vi "Locate P2t.vi"(4 "Template File Path (Locate P2 Hole)":path=path "C:/Users/serce/Desktop/Smart Vision System Testbench/P2/P2 Hole Template.png", 6 "Error In":errorcluster, 9 "Image In":T1) -> (0 "Error Out":errorcluster, 1 "Bounding Box":cluster{"x":sgl, "y":sgl}[](array[cluster]), 3 "Image Out":T1, 5 "Number of Matches (Locate P2 Hole)":i32)   [LabVIEW 2020]
uses:
  <vilib>/vision/Image Controls.llb/IMAQ Image.ctl
  <vilib>/vision/Pattern Matching.llb/IMAQ Curve Parameters.ctl
  <vilib>/vision/Pattern Matching.llb/IMAQ Match Range Setting.ctl
  <vilib>/vision/Pattern Matching.llb/IMAQ Geometric Pattern 2 Advanced Match Options.ctl
  <vilib>/vision/Image Controls.llb/Vision Info Type2.ctl
  <vilib>/vision/NI_Vision_Development_Module.lvlib
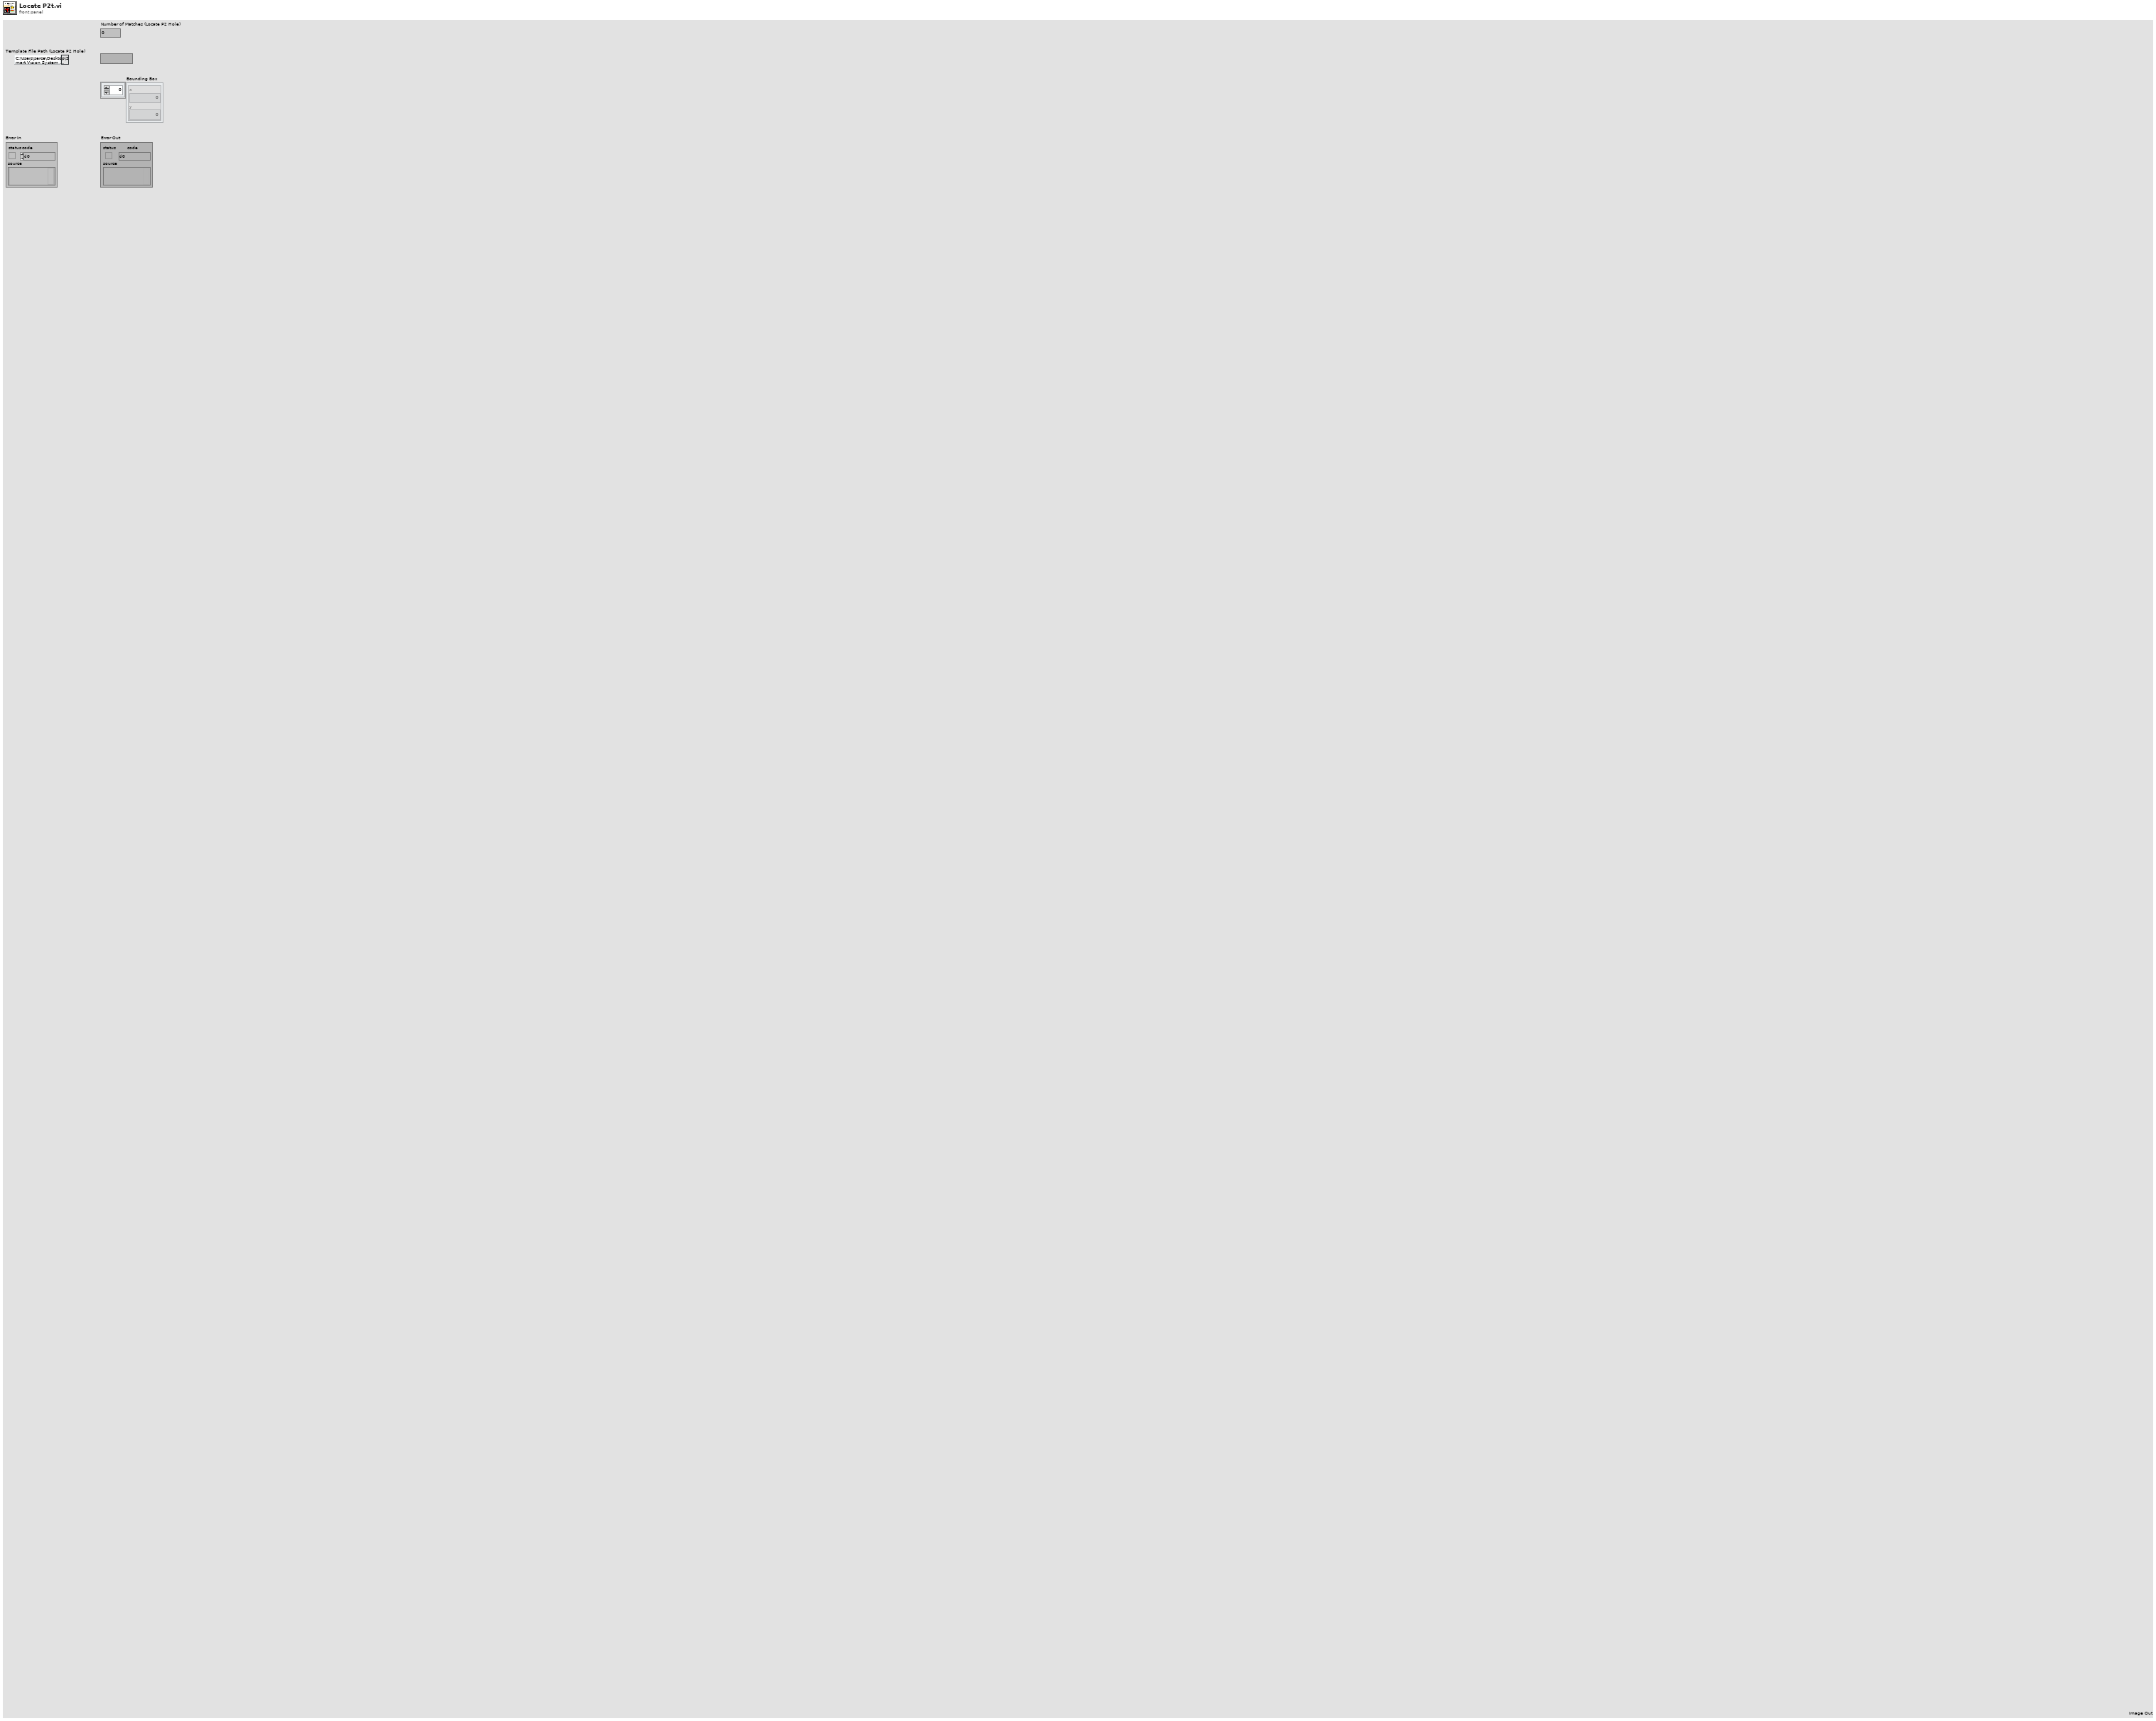
[diagram p1: front panel]
types:
  T1 = typedef "IMAQ Image.ctl" = refnum<image>
  T2 = cluster{"Origin Pixel":cluster{"X":sgl, "Y":sgl}, "X Axis Pixel":cluster{"X":sgl, "Y":sgl}, "Axis Reference":u32}
  T3 = typedef "Vision Info Type2.ctl" = u32
  T4 = typedef "Simple Grid Descriptor" = cluster{"X Step":sgl, "Y Step":sgl, "Unit":T5}
  T5 = typedef "Image Unit" = enum32{"Undefined", "Angström", "Micrometer", "Millimeter", "Centimeter", "Meter", "Kilometer", "Microinch", "Inch", "Feet", "Nautical miles", "Standard miles", "Steps"}
  T6 = enum16{"Reset", "Update Coordinate System", "Get Coordinate System"}
  T7 = enum16{"Horizontal Motion", "Vertical Motion", "Horizontal and Vertical Motion", "Horizontal, Vertical and Angular Motion"}
  T8 = cluster{"Origin":cluster{"X":sgl, "Y":sgl}, "Angle (deg)":sgl, "Axis Reference":u32}
  T9 = typedef "IMAQ Curve Parameters.ctl" = cluster{"Extraction Mode":u32, "Edge Threshold":i32, "Edge Filter Size":u32, "Min Length":i32, "Row Search Step Size":i32, "Col Search Step Size":i32, "Max Endpoint Gap":i32, "Closed":bool, "Subpixel":bool}
  T10 = typedef "IMAQ Match Range Setting.ctl" = cluster{"Match Constraints":u32, "Min":dbl, "Max":dbl}
  T11 = typedef "IMAQ Geometric Pattern 2 Advanced Match Options.ctl" = u16
  T12 = cluster{"Curve Parameters":T9, "Match Mode":cluster{"Rotation":bool, "Scale":bool, "Occlusion":bool, "Reserved 1":bool, "Reserved 2":bool, "Reserved 3":bool}, "Range Settings":T10[], "Number of Matches":i32, "Minimum Match Score":sgl, "SubPixel Accuracy":bool, "Adv. Geometric Match Options 2":cluster{"Setup Data Item":T11, "Item Value":dbl}[]}
  T13 = cluster{"Global Rectangle":i32[], "Contours":cluster{"ID":enum32{"External", "Internal"}, "Type":u32, "Coordinates":i32[]}[]}
  T14 = cluster{"Brightness":sgl, "Contrast":sgl, "Gamma":sgl}
  T15 = typedef "IMAQ GM Match Report.ctl" = cluster{"Position":cluster{"x":sgl, "y":sgl}, "Angle":sgl, "Scale":sgl, "Score":sgl, "Bounding Box":cluster{"x":sgl, "y":sgl}[], "Contrast Reversed":bool, "Occlusion %":sgl, "Template Target Curve Score":sgl, "Target Template Curve Score":sgl, "Correlation Score":sgl}
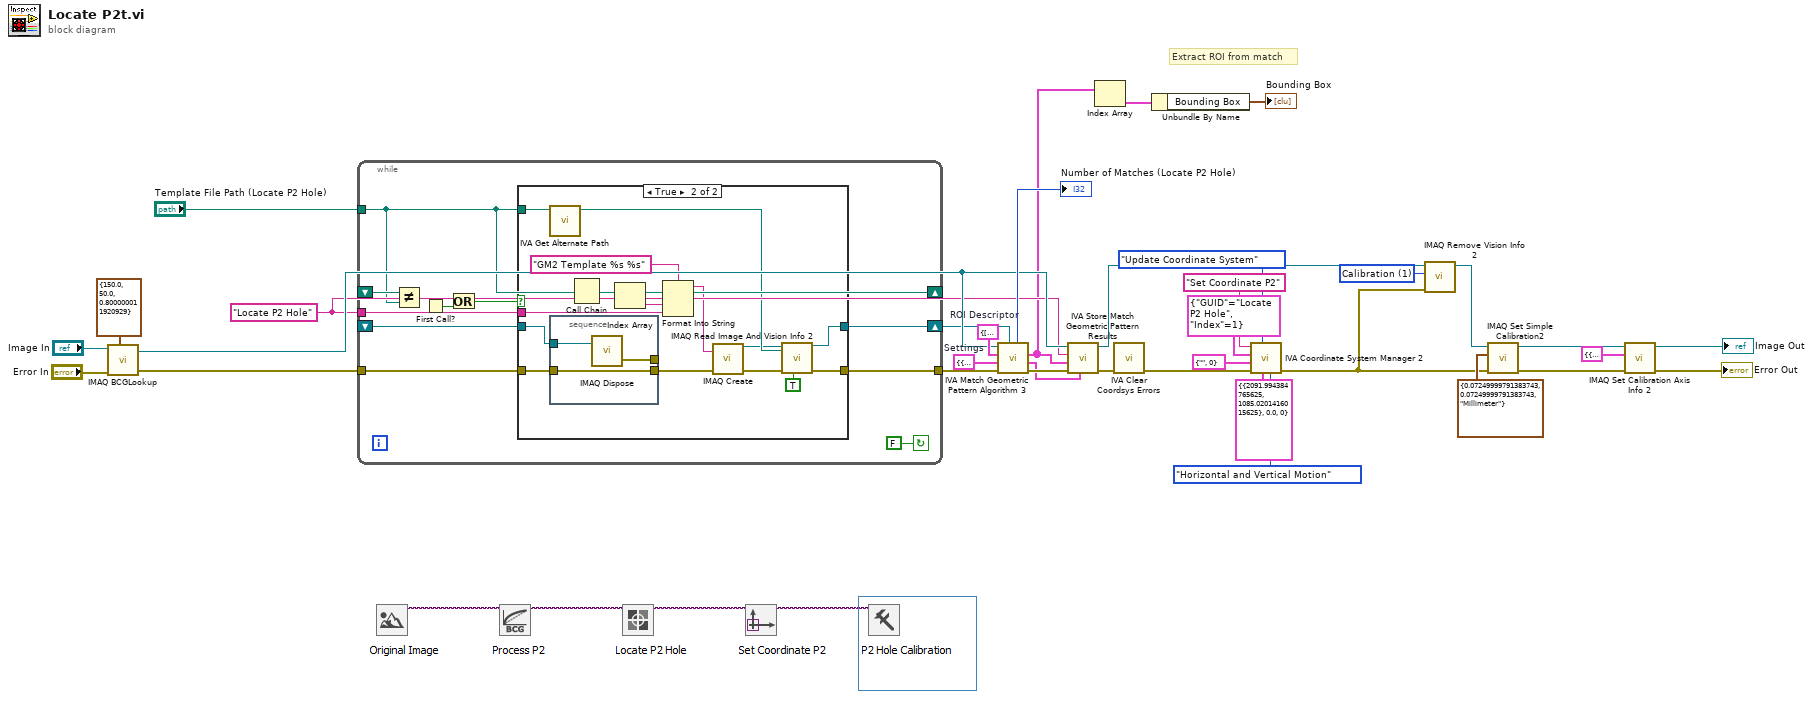
[diagram p0: block diagram]
diagram:
  w12 = T3 1 items=["Any", "Calibration", "Overlay", "Grayscale Template", "Color Template", "Geometric Template", "Custom Data", "Golden Template", "Geometric Template 2", "Contour Data", "Camera Model"] ("Vision Info")
  w25 = T12 {"Curve Parameters"={"Extraction Mode"=0, "Edge Threshold"=50, "Edge Filter Size"=1, "Min Length"=25, "Row Search Step Size"=15, "Col Search Step Size"=15, "Max Endpoint Gap"=10, "Closed"=FALSE, "Subpixel"=FALSE}, "Match Mode"={"Rotation"=TRUE, "Scale"=FALSE, "Occlusion"=FALSE, "Reserved 1"=FALSE, "Reserved 2"=FALSE, "Reserved 3"=FALSE}, "Range Settings"=[{"Match Constraints"=0, "Min"=-5.0, "Max"=5.0}], "Number of Matches"=1, "Minimum Match Score"=800.0, "SubPixel Accuracy"=TRUE, "Adv. Geometric Match Options 2"=[{"Setup Data Item"=0, "Item Value"=0.0}, {"Setup Data Item"=1, "Item Value"=50.0}, {"Setup Data Item"=2, "Item Value"=1.0}, {"Setup Data Item"=3, "Item Value"=25.0}, {"Setup Data Item"=4, "Item Value"=15.0}, {"Setup Data Item"=5, "Item Value"=15.0}, {"Setup Data Item"=6, "Item Value"=10.0}, {"Setup Data Item"=7, "Item Value"=0.0}, {"Setup Data Item"=8, "Item Value"=0.0}, {"Setup Data Item"=9, "Item Value"=1.0}, {"Setup Data Item"=14, "Item Value"=0.0}]}  # Settings
  w24 = "Locate P2 Hole" ("Step Name")
  w31 = T13 {"Global Rectangle"=[20, 20, 3980, 2219], "Contours"=[{"ID"=enum."External", "Type"=3, "Coordinates"=[20, 20, 3980, 2219]}]}  # ROI Descriptor
  # "Extract ROI from match"
  n1 = call "IMAQ BCGLookup"("Image Src"="Image In", "BCG Values"=T14 {"Brightness"=150.0, "Contrast"=50.0, "Gamma"=0.8}, "error in (no error)"="Error In") -> ("Image Dst Out"=w26:T1, "error out"=w27:errorcluster)  [unwired: 2 in, 2 out]
  n2 = while {
    shift-right: [w46] -> w22
    shift-left: _ -> [w45]
    tunnel: [w43] -> w23
    tunnel: w27 -> [w42]
    tunnel: "Template File Path (Locate P2 Hole)" -> [w36]
    tunnel: w24 -> [w41]
    shift-right: [w36] -> _
    shift-left: _ -> [w37]
    stop <- FALSE continue-if-true
    n3 = Not Equal?(x=w37, y=w36) -> (x != y?=w39:bool)
    n4 = First Call?() -> (First Call?: T/F=w40:bool)
    n5 = Or(x=w39, y=w40) -> (x .or. y?=w38:bool)
    n6 = case shown="True" w38 {
      tunnel: [w48 w50] -> w46
      tunnel: w45 -> [w48 w57]
      tunnel: [w47 w52] -> w43
      tunnel: w42 -> [w47 w58]
      tunnel: w41 -> [_ w59]
      tunnel: w36 -> [_ w56]
      frame False {
      }
      frame True {
        n7 = call <vilib>:"IVA Get Alternate Path.vi"("Path In"=w56) -> ("Path Out"=w51:path)  [unwired: 10 out]
        n8 = stacked-sequence {
          tunnel: w58 -> [w66]
          tunnel: w57 -> [w65]
          tunnel: [w66] -> w55
          tunnel: [w64] -> _
          frame #0 {
            n9 = call "IMAQ Dispose"("Image"=w65) -> ("error out"=w64:errorcluster)  [unwired: 2 in, 3 out]
          }
        }
        n10 = Call Chain() -> (call chain=w61:string[])
        n11 = Index Array(array=w61) -> (element=w60:string)  [unwired: 1 in]
        n12 = Format Into String(format string="GM2 Template %s %s" ("Image Name"), w60, w59) -> (resulting string=w63:string)  [unwired: 2 in, 1 out]
        n13 = call "IMAQ Create"("Image Name"=w63, "error in (no error)"=w55) -> ("New Image"=w49:T1, "error out"=w53:errorcluster)  [unwired: 2 in, 1 out]
        n14 = call "IMAQ Read Image And Vision Info 2"("Use File Path Image Type"=TRUE, "File Path"=w51, "error in (no error)"=w53, "Image"=w49) -> ("error out"=w52:errorcluster, "Image Out"=w50:T1)  [unwired: 5 in, 1 out]
      }
    }
  }
  n15 = call <vilib>:"IVA Match Geometric Pattern Algorithm 3.vi"("Template"=w22, "error in (no error)"=w23, "Settings"=w25, "ROI Descriptor"=w31, "Image"=w26) -> ("error out"=w30:errorcluster, "Calibrated Matches"=w29:T15[], "Matches"=w2:T15[], "Number of Matches"=→"Number of Matches (Locate P2 Hole)":i32)  [unwired: 3 out]
  n16 = call <vilib>:"IVA Store Match Geometric Pattern Results.vi"("Calibrated Matches"=w29, "error in (no error)"=w30, "Matches"=w2, "Step Name"=w24, "Image in"=w26) -> ("error out"=w21:errorcluster, "Image dup"=w11:T1)  [unwired: 5 out]
  n17 = Index Array(array=w2) -> (element=w3:T15)  [unwired: 1 in]
  n18 = call <vilib>:"IVA Clear Coordsys Errors.vi"("error in (no error)"=w21) -> ("error out"=w14:errorcluster)  [unwired: 10 in]
  n19 = Unbundle By Name(w3) -> ("Bounding Box"=→"Bounding Box":cluster{"x":sgl, "y":sgl}[])
  n20 = call <vilib>:"IVA Coordinate System Manager 2.vi"("Mode"=T7."Horizontal and Vertical Motion", "Reference System"=T8 {"Origin"={"X"=2091.9944, "Y"=1085.0201}, "Angle (deg)"=0.0, "Axis Reference"=0}, "Function"=T6."Update Coordinate System", "error in (no error)"=w14, "Angle ID"=cluster{"GUID":string, "Index":i32} {"GUID"="", "Index"=0}, "Origin ID"=cluster{"GUID":string, "Index":i32} {"GUID"="Locate P2 Hole", "Index"=1}, "Coordinate System Name"="Set Coordinate P2") -> ("error out"=w9:errorcluster)  [unwired: 4 out]
  n21 = call "IMAQ Remove Vision Info 2"("error in (no error)"=w9, "Vision Info"=w12, "Image"=w11) -> ("Image Out"=w10:T1)  [unwired: 8 out]
  n22 = call "IMAQ Set Simple Calibration2"("error in (no error)"=w9, "Pixel Distances"=T4 {"X Step"=0.0725, "Y Step"=0.0725, "Unit"=enum."Millimeter"} ("Grid Descriptor"), "Image"=w10) -> ("error out"=w5:errorcluster, "Calibration Template Image"=w6:T1)  [unwired: 2 in, 5 out]
  n23 = call-poly "IMAQ Set Calibration Axis Info 2"("error in (no error)"=w5, "Calibration Axis Info"=T2 {"Origin Pixel"={"X"=1990.0, "Y"=1085.0}, "X Axis Pixel"={"X"=2040.0, "Y"=1085.0}, "Axis Reference"=1}, "Calibration Template Image In"=w6) -> ("error out"=→"Error Out":errorcluster, "Calibration Template Image Out"=→"Image Out":T1)  [unwired: 7 out]
